vi "Latch.vi"(8 "Reset":bool, 11 "Set":bool) -> (1 "Out":bool)   [LabVIEW 2013, in "ProcessorHelperFunctions.lvlib"]
uses:
  ProcessorHelperFunctions.lvlib
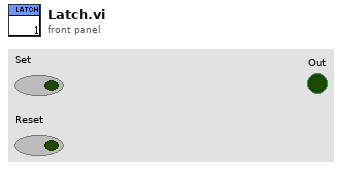
[diagram p1: front panel]
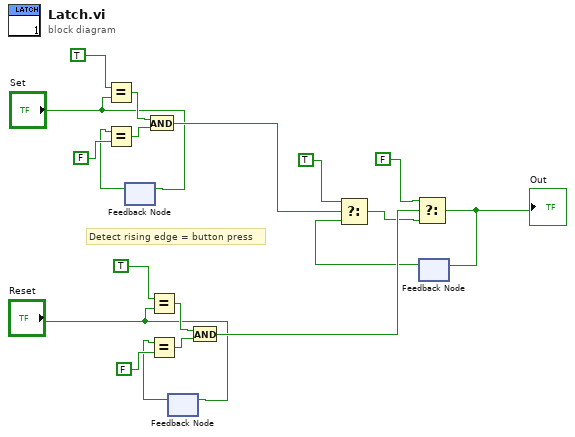
[diagram p0: block diagram]
diagram:
  # "Detect rising edge = button press"
  n1 = Equal?(x=TRUE, y="Set") -> (x = y?=w15:bool)
  n2 = feedback-in #1("Set") -> ()
  n3 = feedback #1() -> (w18:bool)  [unwired: 1 in]
  n4 = Equal?(x=w18, y=FALSE) -> (x = y?=w16:bool)
  n5 = And(x=w15, y=w16) -> (x .and. y?=w9:bool)
  n6 = Equal?(x=TRUE, y="Reset") -> (x = y?=w10:bool)
  n7 = feedback #2() -> (w13:bool)  [unwired: 1 in]
  n8 = Equal?(x=w13, y=FALSE) -> (x = y?=w11:bool)
  n9 = feedback-in #2("Reset") -> ()
  n10 = And(x=w10, y=w11) -> (x .and. y?=w8:bool)
  n11 = feedback #3() -> (w4:bool)  [unwired: 1 in]
  n12 = Select(t=TRUE, s=w9, f=w4) -> (s? t:f=w7:bool)
  n13 = Select(t=FALSE, s=w8, f=w7) -> (s? t:f=w5:bool)
  "Out" <- w5
  n14 = feedback-in #3(w5) -> ()
